vi "WPI_CANJaguar_GetOutput.vi"(8 "error in (no error)":errorcluster, 11 "MotorControlDevRef":T1={"DeviceStatus"={"status"=FALSE, "code"=0, "source"=""}, "Type"=enum."PWM", "PWM"={"PWM Channel"=enum."Invalid", "DeadBand"={"Name"="", "maxPositivePwm"=0, "minPositivePwm"=0, "centerPwm"=0, "maxNegativePwm"=0, "minNegativePwm"=0, "angularRange"=0}}, "CAN"={"Device Number"=0, "SetOutput VI Ref"=variant(enum8{"Percent VBus", "Current", "Speed", "Position", "Voltage"} enum."Percent VBus"), "GetOutput VI Ref"=variant(refnum<k1> refnum), "Enable VI Ref"=variant(dbl 12.0), "Disable VI Ref"=variant(enum8{"Percent VBus", "Speed", "Position", "Slave", "Unchanged / Invalid", "Voltage Compensation", "Current", "Motion Profile"} enum."Percent VBus"), "Data"=variant}, "Invert"=FALSE}) -> (0 "error out":errorcluster, 2 "Output":dbl, 3 "MotorControlDevRef":T1={"DeviceStatus"={"status"=FALSE, "code"=0, "source"=""}, "Type"=enum."PWM", "PWM"={"PWM Channel"=enum."Invalid", "DeadBand"={"Name"="", "maxPositivePwm"=0, "minPositivePwm"=0, "centerPwm"=0, "maxNegativePwm"=0, "minNegativePwm"=0, "angularRange"=0}}, "CAN"={"Device Number"=0, "SetOutput VI Ref"=variant(enum8{"Percent VBus", "Current", "Speed", "Position", "Voltage"} enum."Percent VBus"), "GetOutput VI Ref"=variant(refnum<k1> refnum), "Enable VI Ref"=variant(dbl 12.0), "Disable VI Ref"=variant(enum8{"Percent VBus", "Speed", "Position", "Slave", "Unchanged / Invalid", "Voltage Compensation", "Current", "Motion Profile"} enum."Percent VBus"), "Data"=variant}, "Invert"=FALSE})   [LabVIEW 2016]
doc: "Returns the last output value or set-point that was written to the motor controller with the <B>Set Output</B> VI."
uses:
  <vilib>/Rock Robotics/WPI/MotorControl/WPI_MotorControlDeviceRef.ctl
  <vilib>/Rock Robotics/WPI/MotorControl/WPI_MotorControlType.ctl
  <vilib>/Rock Robotics/SystemInterfaces/DIO/FPGA_DIOPWMChannel.ctl
  <vilib>/Rock Robotics/WPI/PWM/WPI_PWMDeadband.ctl
  <vilib>/Rock Robotics/WPI/ThirdParty/CanMotor/CAN Jaguar/SubVIs/WPI_CANJaguar_RefNumData.ctl
  <vilib>/Rock Robotics/WPI/ThirdParty/CanMotor/CAN Jaguar/SubVIs/WPI_CANJaguar_ControlMode.ctl
  <vilib>/Rock Robotics/WPI/ThirdParty/CanMotor/CAN Jaguar/SubVIs/WPI_CAN_MotorMessageIDs.ctl
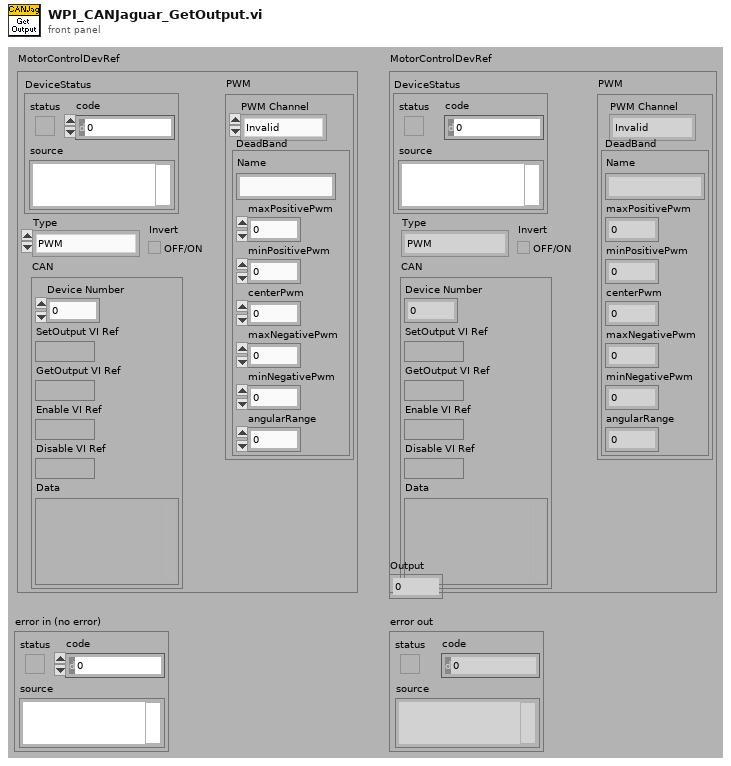
[diagram p1: front panel]
types:
  T1 = typedef "WPI_MotorControlDeviceRef.ctl" = cluster{"DeviceStatus":errorcluster, "Type":T2, "PWM":cluster{"PWM Channel":T3, "DeadBand":T4}, "CAN":cluster{"Device Number":u8, "SetOutput VI Ref":variant, "GetOutput VI Ref":variant, "Enable VI Ref":variant, "Disable VI Ref":variant, "Data":variant}, "Invert":bool}
  T2 = typedef "WPI_MotorControlType.ctl" = enum16{"PWM", "CAN"}
  T3 = typedef "FPGA_DIOPWMChannel.ctl" = enum8{"PWM 0", "PWM 1", "PWM 2", "PWM 3", "PWM 4", "PWM 5", "PWM 6", "PWM 7", "PWM 8", "PWM 9", "PWM MXP 0", "PWM MXP 1", "PWM MXP 2", "PWM MXP 3", "PWM MXP 4", "PWM MXP 5", "PWM MXP 6", "PWM MXP 7", "PWM MXP 8", "PWM MXP 9", "Invalid"}
  T4 = typedef "WPI_PWMDeadband.ctl" = cluster{"Name":string, "maxPositivePwm":i32, "minPositivePwm":i32, "centerPwm":i32, "maxNegativePwm":i32, "minNegativePwm":i32, "angularRange":u16}
  T5 = typedef "WPI_CANJaguar_RefNumData.ctl" = cluster{"CAN.Max Vout":dbl, "Control Mode":T6, "semaphore":T7}
  T6 = typedef "WPI_CANJaguar_ControlMode.ctl" = enum8{"Percent VBus", "Current", "Speed", "Position", "Voltage"}
  T7 = typedef "Semaphore RefNum" = refnum<k1>
  T8 = enum16{"big-endian, network order", "native, host order", "little-endian"}
  T9 = typedef "WPI_CAN_MotorMessageIDs.ctl" = u32
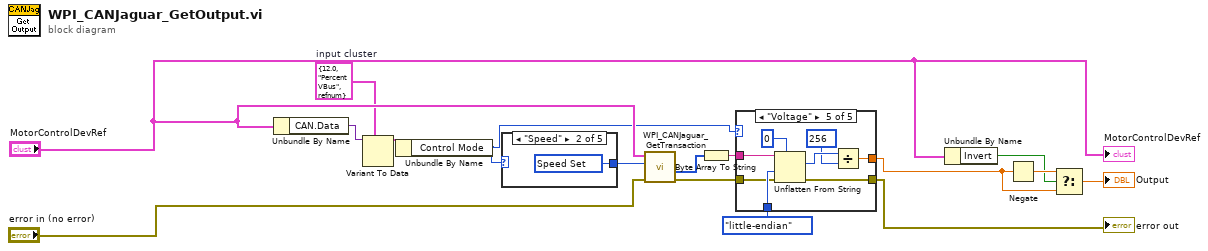
[diagram p0: block diagram]
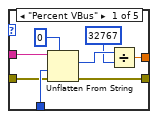
[diagram p2: hidden frame]
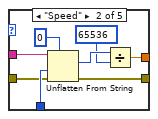
[diagram p3: hidden frame]
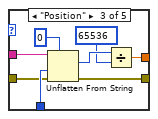
[diagram p4: hidden frame]
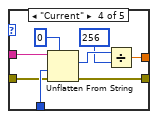
[diagram p5: hidden frame]
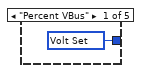
[diagram p6: hidden frame]
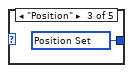
[diagram p7: hidden frame]
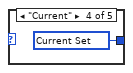
[diagram p8: hidden frame]
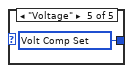
[diagram p9: hidden frame]
diagram:
  w3 = T5 {"CAN.Max Vout"=12.0, "Control Mode"=enum."Percent VBus", "semaphore"=refnum}  # input cluster
  n1 = Unbundle By Name("MotorControlDevRef") -> ("CAN.Data"=w4:variant)
  n2 = Variant To Data(type=w3, Variant=w4) -> (data=w2:T5)  [unwired: 1 in, 1 out]
  n3 = Unbundle By Name(w2) -> ("Control Mode"=w1:T6)
  n4 = case shown="\"Position\"" w1 {
    tunnel: [w17 w18 w19 w20 w21] -> w9
    frame "Percent VBus" {
      w17 = T9 33685632 items=["Volt Enable"=33685504, "Volt Disable"=33685568, "Volt Set"=33685632, "Volt Set Ramp"=33685696, "Volt Set No Ack"=33686080, "Speed Enable"=33686528, "Speed Disable"=33686592, "Speed Set"=33686656, "Speed P"=33686720, "Speed I"=33686784, "Speed D"=33686848, "Speed Ref"=33686912, "Speed Set No Ack"=33687232, "Volt Comp Enable"=33687552, "Volt Comp Disable"=33687616, "Volt Comp Set"=33687680, "Volt Comp In Ramp"=33687744, "Volt Comp Comp Ramp"=33687808, "Volt Comp Set No Ack"=33688128, "Position Enable"=33688576, "Position Disable"=33688640, "Position Set"=33688704, "Position P"=33688768, "Position I"=33688832, "Position D"=33688896, "Position Ref"=33688960, "Position Set No Ack"=33689280, "Current Enable"=33689600, "Current Disable"=33689664, "Current Set"=33689728, "Current P"=33689792, "Current I"=33689856, "Current D"=33689920, "Current Set No Ack"=33690240, "Status Percent VBus"=33690624, "Status VBus"=33690688, "Status Current"=33690752, "Status Temp"=33690816, "Status Position"=33690880, "Status Speed"=33690944, "Status Limit"=33691008, "Status Fault"=33691072, "Status Power"=33691136, "Status Control Mode"=33691200, "Status VOut"=33691264, "Status Sticky Fault"=33691328, "Status Fault Count"=33691392, "Periodic Status Enable 0"=33691648, "Periodic Status Enable 1"=33691712, "Periodic Status Enable 2"=33691776, "Periodic Status Enable 3"=33691840, "Periodic Status Config 0"=33691904, "Periodic Status Config 1"=33691968, "Periodic Status Config 2"=33692032, "Periodic Status Config 3"=33692096, "Periodic Status Data 0"=33692160, "Periodic Status Data 1"=33692224, "Periodic Status Data 2"=33692288, "Periodic Status Data 3"=33692352, "Config Num Brushes"=33692672, "Config Encoder Lines"=33692736, "Config Pot Turns"=33692800, "Config Brake Coast"=33692864, "Config Limit Mode"=33692928, "Config Limit Fwd"=33692992, "Config Limit Rev"=33693056, "Config Max VOut"=33693120, "Config Fault Time"=33693184, "Motor Ack"=33693696] ("CAN Motor Message IDs")
    }
    frame "Speed" {
      w18 = T9 33686656 items=["Volt Enable"=33685504, "Volt Disable"=33685568, "Volt Set"=33685632, "Volt Set Ramp"=33685696, "Volt Set No Ack"=33686080, "Speed Enable"=33686528, "Speed Disable"=33686592, "Speed Set"=33686656, "Speed P"=33686720, "Speed I"=33686784, "Speed D"=33686848, "Speed Ref"=33686912, "Speed Set No Ack"=33687232, "Volt Comp Enable"=33687552, "Volt Comp Disable"=33687616, "Volt Comp Set"=33687680, "Volt Comp In Ramp"=33687744, "Volt Comp Comp Ramp"=33687808, "Volt Comp Set No Ack"=33688128, "Position Enable"=33688576, "Position Disable"=33688640, "Position Set"=33688704, "Position P"=33688768, "Position I"=33688832, "Position D"=33688896, "Position Ref"=33688960, "Position Set No Ack"=33689280, "Current Enable"=33689600, "Current Disable"=33689664, "Current Set"=33689728, "Current P"=33689792, "Current I"=33689856, "Current D"=33689920, "Current Set No Ack"=33690240, "Status Percent VBus"=33690624, "Status VBus"=33690688, "Status Current"=33690752, "Status Temp"=33690816, "Status Position"=33690880, "Status Speed"=33690944, "Status Limit"=33691008, "Status Fault"=33691072, "Status Power"=33691136, "Status Control Mode"=33691200, "Status VOut"=33691264, "Status Sticky Fault"=33691328, "Status Fault Count"=33691392, "Periodic Status Enable 0"=33691648, "Periodic Status Enable 1"=33691712, "Periodic Status Enable 2"=33691776, "Periodic Status Enable 3"=33691840, "Periodic Status Config 0"=33691904, "Periodic Status Config 1"=33691968, "Periodic Status Config 2"=33692032, "Periodic Status Config 3"=33692096, "Periodic Status Data 0"=33692160, "Periodic Status Data 1"=33692224, "Periodic Status Data 2"=33692288, "Periodic Status Data 3"=33692352, "Config Num Brushes"=33692672, "Config Encoder Lines"=33692736, "Config Pot Turns"=33692800, "Config Brake Coast"=33692864, "Config Limit Mode"=33692928, "Config Limit Fwd"=33692992, "Config Limit Rev"=33693056, "Config Max VOut"=33693120, "Config Fault Time"=33693184, "Motor Ack"=33693696] ("CAN Motor Message IDs")
    }
    frame "Position" {
      w19 = T9 33688704 items=["Volt Enable"=33685504, "Volt Disable"=33685568, "Volt Set"=33685632, "Volt Set Ramp"=33685696, "Volt Set No Ack"=33686080, "Speed Enable"=33686528, "Speed Disable"=33686592, "Speed Set"=33686656, "Speed P"=33686720, "Speed I"=33686784, "Speed D"=33686848, "Speed Ref"=33686912, "Speed Set No Ack"=33687232, "Volt Comp Enable"=33687552, "Volt Comp Disable"=33687616, "Volt Comp Set"=33687680, "Volt Comp In Ramp"=33687744, "Volt Comp Comp Ramp"=33687808, "Volt Comp Set No Ack"=33688128, "Position Enable"=33688576, "Position Disable"=33688640, "Position Set"=33688704, "Position P"=33688768, "Position I"=33688832, "Position D"=33688896, "Position Ref"=33688960, "Position Set No Ack"=33689280, "Current Enable"=33689600, "Current Disable"=33689664, "Current Set"=33689728, "Current P"=33689792, "Current I"=33689856, "Current D"=33689920, "Current Set No Ack"=33690240, "Status Percent VBus"=33690624, "Status VBus"=33690688, "Status Current"=33690752, "Status Temp"=33690816, "Status Position"=33690880, "Status Speed"=33690944, "Status Limit"=33691008, "Status Fault"=33691072, "Status Power"=33691136, "Status Control Mode"=33691200, "Status VOut"=33691264, "Status Sticky Fault"=33691328, "Status Fault Count"=33691392, "Periodic Status Enable 0"=33691648, "Periodic Status Enable 1"=33691712, "Periodic Status Enable 2"=33691776, "Periodic Status Enable 3"=33691840, "Periodic Status Config 0"=33691904, "Periodic Status Config 1"=33691968, "Periodic Status Config 2"=33692032, "Periodic Status Config 3"=33692096, "Periodic Status Data 0"=33692160, "Periodic Status Data 1"=33692224, "Periodic Status Data 2"=33692288, "Periodic Status Data 3"=33692352, "Config Num Brushes"=33692672, "Config Encoder Lines"=33692736, "Config Pot Turns"=33692800, "Config Brake Coast"=33692864, "Config Limit Mode"=33692928, "Config Limit Fwd"=33692992, "Config Limit Rev"=33693056, "Config Max VOut"=33693120, "Config Fault Time"=33693184, "Motor Ack"=33693696] ("CAN Motor Message IDs")
    }
    frame "Current" {
      w20 = T9 33689728 items=["Volt Enable"=33685504, "Volt Disable"=33685568, "Volt Set"=33685632, "Volt Set Ramp"=33685696, "Volt Set No Ack"=33686080, "Speed Enable"=33686528, "Speed Disable"=33686592, "Speed Set"=33686656, "Speed P"=33686720, "Speed I"=33686784, "Speed D"=33686848, "Speed Ref"=33686912, "Speed Set No Ack"=33687232, "Volt Comp Enable"=33687552, "Volt Comp Disable"=33687616, "Volt Comp Set"=33687680, "Volt Comp In Ramp"=33687744, "Volt Comp Comp Ramp"=33687808, "Volt Comp Set No Ack"=33688128, "Position Enable"=33688576, "Position Disable"=33688640, "Position Set"=33688704, "Position P"=33688768, "Position I"=33688832, "Position D"=33688896, "Position Ref"=33688960, "Position Set No Ack"=33689280, "Current Enable"=33689600, "Current Disable"=33689664, "Current Set"=33689728, "Current P"=33689792, "Current I"=33689856, "Current D"=33689920, "Current Set No Ack"=33690240, "Status Percent VBus"=33690624, "Status VBus"=33690688, "Status Current"=33690752, "Status Temp"=33690816, "Status Position"=33690880, "Status Speed"=33690944, "Status Limit"=33691008, "Status Fault"=33691072, "Status Power"=33691136, "Status Control Mode"=33691200, "Status VOut"=33691264, "Status Sticky Fault"=33691328, "Status Fault Count"=33691392, "Periodic Status Enable 0"=33691648, "Periodic Status Enable 1"=33691712, "Periodic Status Enable 2"=33691776, "Periodic Status Enable 3"=33691840, "Periodic Status Config 0"=33691904, "Periodic Status Config 1"=33691968, "Periodic Status Config 2"=33692032, "Periodic Status Config 3"=33692096, "Periodic Status Data 0"=33692160, "Periodic Status Data 1"=33692224, "Periodic Status Data 2"=33692288, "Periodic Status Data 3"=33692352, "Config Num Brushes"=33692672, "Config Encoder Lines"=33692736, "Config Pot Turns"=33692800, "Config Brake Coast"=33692864, "Config Limit Mode"=33692928, "Config Limit Fwd"=33692992, "Config Limit Rev"=33693056, "Config Max VOut"=33693120, "Config Fault Time"=33693184, "Motor Ack"=33693696] ("CAN Motor Message IDs")
    }
    frame "Voltage" {
      w21 = T9 33687680 items=["Volt Enable"=33685504, "Volt Disable"=33685568, "Volt Set"=33685632, "Volt Set Ramp"=33685696, "Volt Set No Ack"=33686080, "Speed Enable"=33686528, "Speed Disable"=33686592, "Speed Set"=33686656, "Speed P"=33686720, "Speed I"=33686784, "Speed D"=33686848, "Speed Ref"=33686912, "Speed Set No Ack"=33687232, "Volt Comp Enable"=33687552, "Volt Comp Disable"=33687616, "Volt Comp Set"=33687680, "Volt Comp In Ramp"=33687744, "Volt Comp Comp Ramp"=33687808, "Volt Comp Set No Ack"=33688128, "Position Enable"=33688576, "Position Disable"=33688640, "Position Set"=33688704, "Position P"=33688768, "Position I"=33688832, "Position D"=33688896, "Position Ref"=33688960, "Position Set No Ack"=33689280, "Current Enable"=33689600, "Current Disable"=33689664, "Current Set"=33689728, "Current P"=33689792, "Current I"=33689856, "Current D"=33689920, "Current Set No Ack"=33690240, "Status Percent VBus"=33690624, "Status VBus"=33690688, "Status Current"=33690752, "Status Temp"=33690816, "Status Position"=33690880, "Status Speed"=33690944, "Status Limit"=33691008, "Status Fault"=33691072, "Status Power"=33691136, "Status Control Mode"=33691200, "Status VOut"=33691264, "Status Sticky Fault"=33691328, "Status Fault Count"=33691392, "Periodic Status Enable 0"=33691648, "Periodic Status Enable 1"=33691712, "Periodic Status Enable 2"=33691776, "Periodic Status Enable 3"=33691840, "Periodic Status Config 0"=33691904, "Periodic Status Config 1"=33691968, "Periodic Status Config 2"=33692032, "Periodic Status Config 3"=33692096, "Periodic Status Data 0"=33692160, "Periodic Status Data 1"=33692224, "Periodic Status Data 2"=33692288, "Periodic Status Data 3"=33692352, "Config Num Brushes"=33692672, "Config Encoder Lines"=33692736, "Config Pot Turns"=33692800, "Config Brake Coast"=33692864, "Config Limit Mode"=33692928, "Config Limit Fwd"=33692992, "Config Limit Rev"=33693056, "Config Max VOut"=33693120, "Config Fault Time"=33693184, "Motor Ack"=33693696] ("CAN Motor Message IDs")
    }
  }
  n5 = call <vilib>:"WPI_CANJaguar_GetTransaction.vi"("error in"="error in (no error)", "Message ID"=w9, "CAN Jaguar Ref"="MotorControlDevRef") -> ("error out"=w8:errorcluster, "Data Out"=w7:u8[])  [unwired: 7 out]
  n6 = Byte Array To String(unsigned byte array=w7) -> (string=w6:string)
  n7 = case shown="\"Voltage\"" w1 {
    tunnel: [w23 w31 w39 w48 w56] -> w12
    tunnel: T8."little-endian" ("byte order (0:big-endian, network order)") -> [w28 w37 w45 w53 w61]
    tunnel: w6 -> [w26 w35 w43 w51 w59]
    tunnel: w8 -> [w25 w34 w42 w50 w58]
    tunnel: [w24 w33 w41 w49 w57] -> w14
    frame "Percent VBus" {
      n8 = Unflatten From String(type=i16 0 ("Voltage"), binary string=w26, byte order (0:big-endian, network order)=w28, error in (no error)=w25) -> (value=w29:i16, error out=w24:errorcluster)  [unwired: 2 out]
      n9 = Divide(x=w29, y=i16 32767) -> (x/y=w23:dbl)
    }
    frame "Speed" {
      n10 = Unflatten From String(type=0 ("Voltage"), binary string=w35, byte order (0:big-endian, network order)=w37, error in (no error)=w34) -> (value=w32:i32, error out=w33:errorcluster)  [unwired: 2 out]
      n11 = Divide(x=w32, y=65536 ("x")) -> (x/y=w31:dbl)
    }
    frame "Position" {
      n12 = Unflatten From String(type=0 ("Voltage"), binary string=w43, byte order (0:big-endian, network order)=w45, error in (no error)=w42) -> (value=w40:i32, error out=w41:errorcluster)  [unwired: 2 out]
      n13 = Divide(x=w40, y=65536 ("x")) -> (x/y=w39:dbl)
    }
    frame "Current" {
      n14 = Unflatten From String(type=i16 0 ("Voltage"), binary string=w51, byte order (0:big-endian, network order)=w53, error in (no error)=w50) -> (value=w47:i16, error out=w49:errorcluster)  [unwired: 2 out]
      n15 = Divide(x=w47, y=i16 256) -> (x/y=w48:dbl)
    }
    frame "Voltage" {
      n16 = Unflatten From String(type=i16 0 ("Voltage"), binary string=w59, byte order (0:big-endian, network order)=w61, error in (no error)=w58) -> (value=w55:i16, error out=w57:errorcluster)  [unwired: 2 out]
      n17 = Divide(x=w55, y=i16 256) -> (x/y=w56:dbl)
    }
  }
  "error out" <- w14
  n18 = Unbundle By Name("MotorControlDevRef") -> ("Invert"=w10:bool)
  n19 = Negate(x=w12) -> (-x=w13:dbl)
  n20 = Select(t=w13, s=w10, f=w12) -> (s? t:f=→"Output":dbl)
  "MotorControlDevRef" <- "MotorControlDevRef"
